vi "MainColorNoise.vi"() -> ()   [LabVIEW 2015]
panel:
  in  "Tab Control 2":T1(tab)
  in  "channel 2":cluster{"output":bool}
  in  "channel 1":T2={"Modulation Waveform (1: Sine)"=200, "modulation"=FALSE, "output"=FALSE, "Peak Deviation (90)"=90.0, "Modulation Frequency (10000)"=10000.0} {"Modulation Waveform (1: Sine)" items=["Sine"=1, "Square"=2, "Triangle"=3, "Ramp Up"=4, "Ramp Down"=5, "Noise"=100, "Arbitrary User1"=200, "Arbitrary User2"=201, "Arbitrary User3"=202, "Arbitrary User4"=203, "Edit Memory"=204]}
  in  "outpout mode":i32(ring) items=["Standard Waveform", "Arbitrary Waveform"]
  in  "configuration main":bool
  in  "amplitude (1)":dbl=0.2
  in  "dc offset (0.00)":dbl
  in  "frequency (1000000)":dbl=80000000.0
  in  "start phase (0.00)":dbl
  in  "amplitude (1) 2":dbl=0.2 caption="amplitude (1)"
  in  "dc offset (0.00) 2":dbl caption="dc offset (0.00)"
  in  "frequency (1000000) 2":dbl=80000000.0 caption="frequency (1000000)"
  in  "start phase (0.00) 2":dbl caption="start phase (0.00)"
  in  "force trigger":bool
  in  "trigger":bool
  in  "trigger source (1: External)":i32(ring)=1 items=["External"=1, "Internal"=3]
  in  "Trigger Slope (1: Positive)":i32(ring)=1 caption="external trigger Slope" items=["Positive"=1, "Negative"=2]
  in  "Output Mode (1: Trigger)":i32(ring)=1 caption="Output Mode" items=["Trigger"=1, "Sync"=2]
  in  "trigger rate (1000.0)":dbl=1000.0 caption="internal trigger rate"
  in  "trigger source (1: External) 2":i32(ring)=1 caption="trigger source (1: External)" items=["External"=1, "Internal"=3]
  in  "Burst Mode (1: Triggered)":i32(ring)=1 items=["Triggered"=1, "Gated"=2]
  in  "loading on slot 2":bool
  in  "slot (0: Slot 1) 2":i32(ring) caption="USER (0: Slot 1)" items=["Slot 1", "Slot 2", "Slot 3", "Slot 4"]
  out "waveform selected":dbl[](graph)
  in  "burst waveform":bool
  out "rep frequency":dbl
  in  "Channel Name (\"1\")":string="1"
  in  "gain (0.5) 2":dbl=0.5 caption="gain"
  out "Noise density":dbl[](graph)
  in  "slot (0: Slot 1)":i32(ring) caption="USER (0: Slot 1)" items=["Slot 1", "Slot 2", "Slot 3", "Slot 4"]
  in  "gain (0.5)":dbl=0.5
  in  "offset (0.00)":dbl
  in  "loading on channel 1":bool
  in  "Waveform Size (1000)":i32=1000
  in  "waveform generation":bool
  out "1/x":dbl
  out "min waveform size":i32
  out "max waveform size":i32
  out "waveform quantum":i32
  out "max number of waveforms":i32
  out "transfer error":errorcluster caption="error out" {"code" format="%.0x"}
  in  "resource name":refnum<k15>
  in  "Stop Button":bool
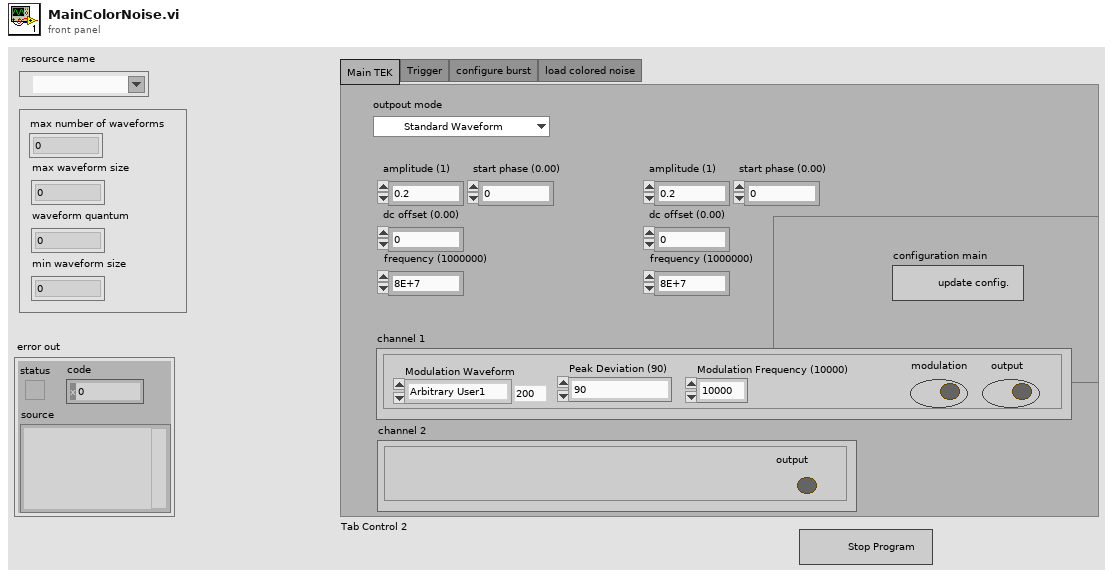
[diagram p1: front panel]
types:
  T1 = enum32{"Main TEK", "Trigger", "configure burst", "load colored noise"}
  T2 = cluster{"Modulation Waveform (1: Sine)":i32, "modulation":bool, "output":bool, "Peak Deviation (90)":dbl, "Modulation Frequency (10000)":dbl}
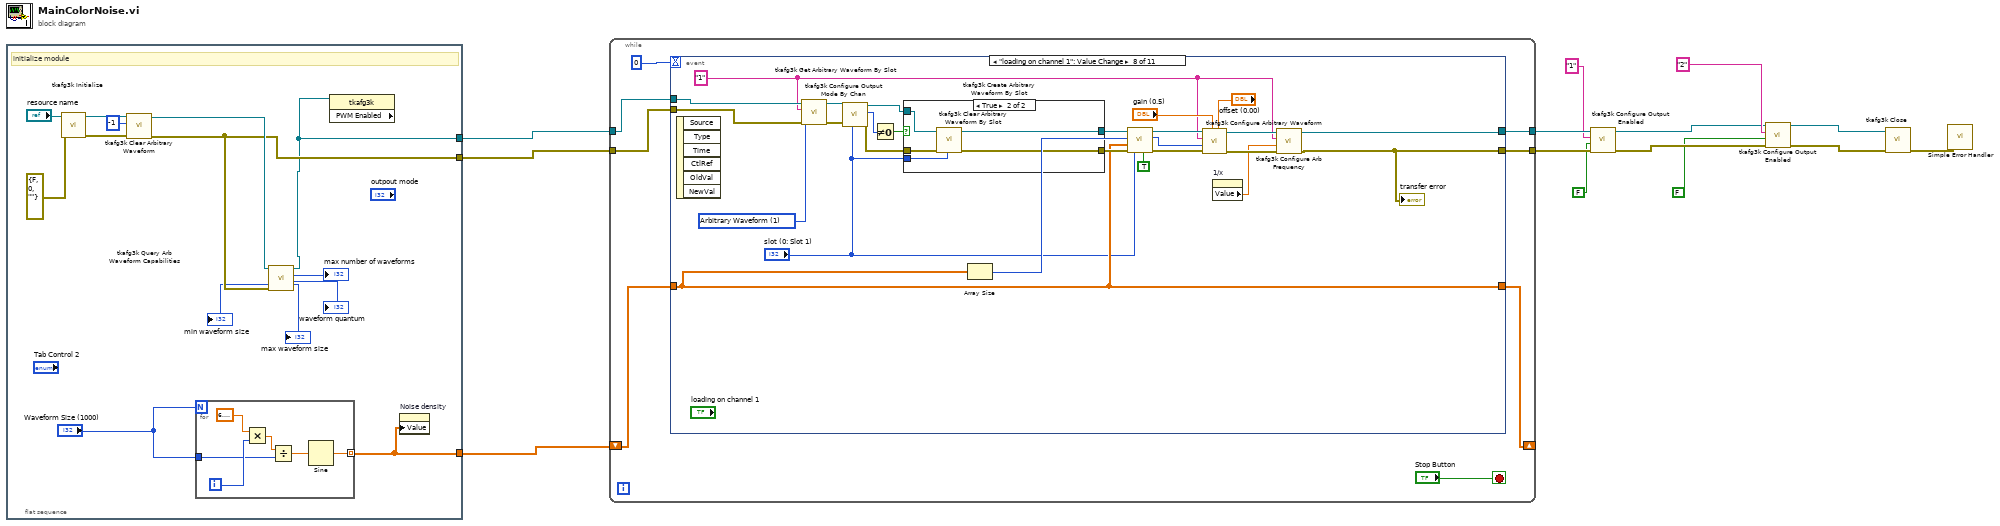
[diagram p0: block diagram]
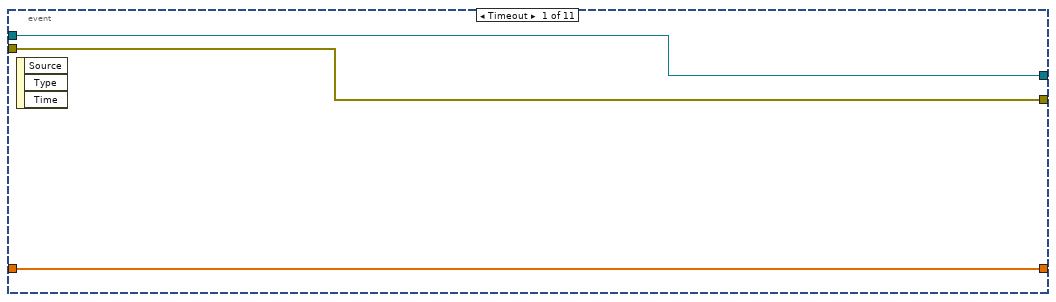
[diagram p2: hidden frame]
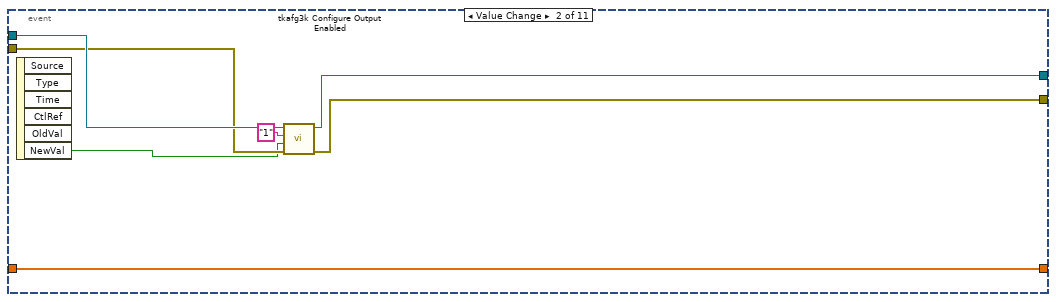
[diagram p3: hidden frame]
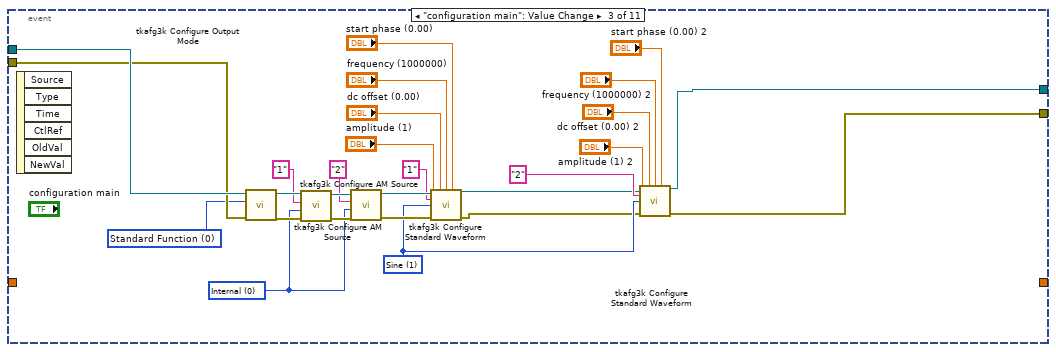
[diagram p4: hidden frame]
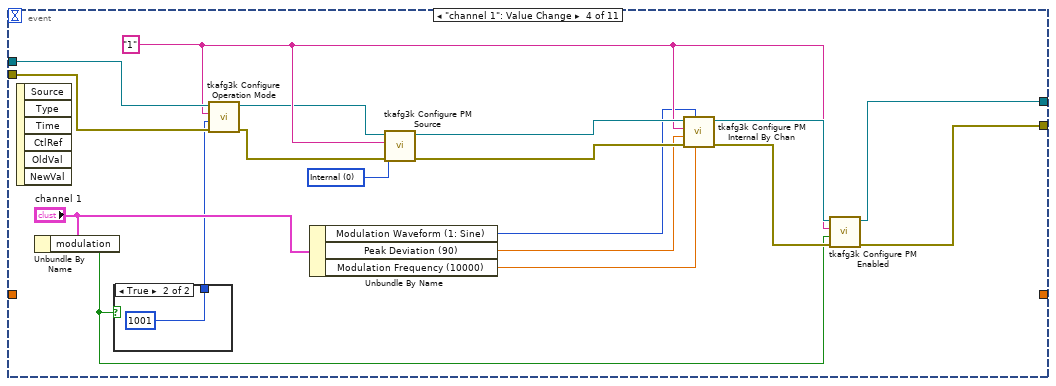
[diagram p5: hidden frame]
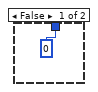
[diagram p6: hidden frame]
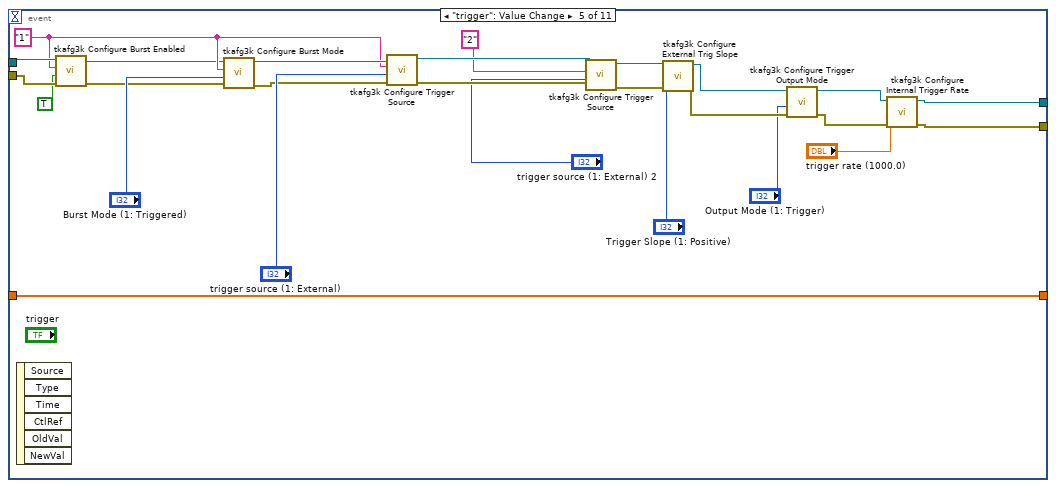
[diagram p7: hidden frame]
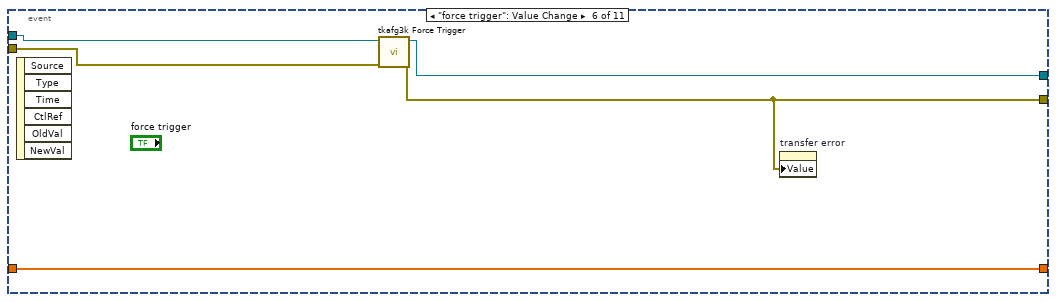
[diagram p8: hidden frame]
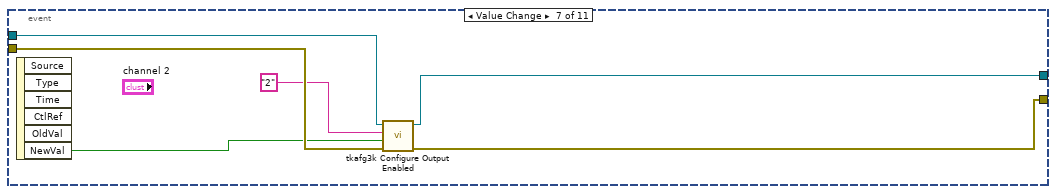
[diagram p9: hidden frame]
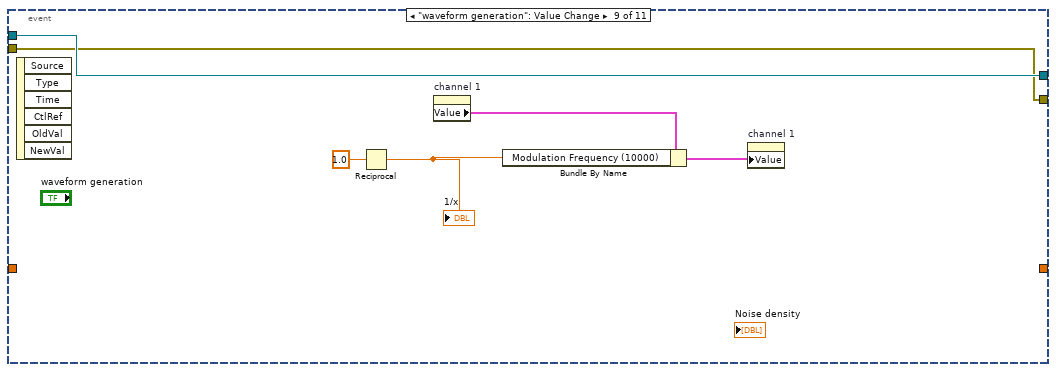
[diagram p11: hidden frame]
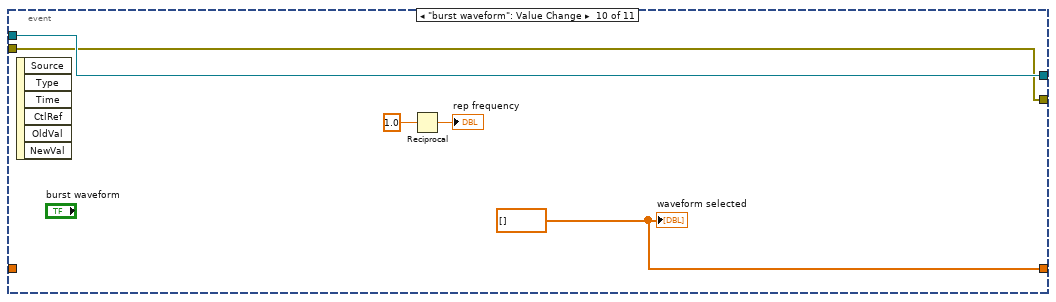
[diagram p12: hidden frame]
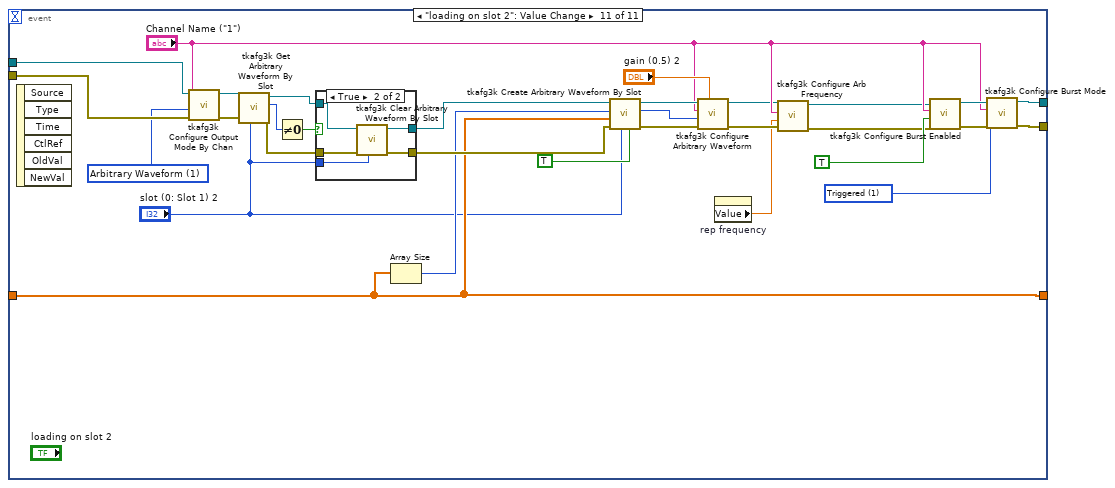
[diagram p13: hidden frame]
diagram:
  n1 = flat-sequence {
    tunnel: [w14] -> w10
    tunnel: [w22] -> w9
    tunnel: [w15] -> w5
    frame #0 {
      # "initialize module"
      n2 = call <instrlib>:"tkafg3k Initialize.vi"("error in (no error)"=errorcluster {"status"=FALSE, "code"=0, "source"=""}, "resource name"="resource name") -> ("error out"=w24:errorcluster, "instrument handle out"=w26:refnum<k15>)  [unwired: 8 in]
      n3 = call <instrlib>:"tkafg3k Clear Arbitrary Waveform.vi"("error in (no error)"=w24, "waveform handle"=-1, "instrument handle"=w26) -> ("error out"=w22:errorcluster, "instrument handle out"=w23:refnum<k15>)  [unwired: 7 in]
      n4 = for {
        N: "Waveform Size (1000)" -> [_]
        tunnel: "Waveform Size (1000)" -> [w29]
        tunnel: [w28] -> w15 mode=indexing
        i -> [w30]
        n5 = Multiply(x=6.283185307179586, y=w30) -> (x*y=w31:dbl)
        n6 = Divide(x=w31, y=w29) -> (x/y=w32:dbl)
        n7 = Sine(x=w32) -> (sin(x)=w28:dbl)
      }
      n8 = call <instrlib>:"tkafg3k Query Arb Waveform Capabilities.vi"("error in (no error)"=w22, "instrument handle"=w23) -> ("waveform quantum"=→"waveform quantum":i32, "max number of waveforms"=→"max number of waveforms":i32, "instrument handle out"=w14:refnum<k15>, "max waveform size"=→"max waveform size":i32, "min waveform size"=→"min waveform size":i32)  [unwired: 4 in, 1 out]
      n9 = property class="tkafg3k" props=["PWM Enabled"](reference=w14) -> ()  [unwired: 1 in, 3 out]
      n10 = property on="Noise density" class="WFGraph (strict)"("Value"=w15) -> ()  [unwired: 2 in, 2 out]
    }
  }
  n11 = while {
    tunnel: w10 -> [w40]
    tunnel: [w39] -> w4
    tunnel: w9 -> [w37]
    tunnel: [w36] -> w8
    shift-right: [w34] -> _
    shift-left: w5 -> [w35]
    stop <- "Stop Button" stop-if-true
    n12 = event shown="[7] \"loading on channel 1\": Value Change" {
      selector: _ -> [_ _ _ _ _ _ _ _ _ _ _]
      dyn-events: _ -> [_ _ _ _ _ _ _ _ _ _ _]
      timeout: 0 -> [_ _ _ _ _ _ _ _ _ _ _]
      tunnel: w40 -> [w43 w51 w78 w96 w104 w129 w135 w154 w174 w179 w204]
      tunnel: [w43 w50 w52 w86 w109 w127 w133 w139 w174 w179 w188] -> w39
      tunnel: w37 -> [w44 w48 w77 w95 w103 w128 w134 w153 w173 w178 w203]
      tunnel: [w44 w47 w53 w85 w108 w125 w132 w140 w173 w178 w189] -> w36
      tunnel: w35 -> [w42 w46 _ _ w124 w126 _ w149 _ _ w198]
      tunnel: [w42 w46 _ _ w124 w126 _ w149 _ w176 w198] -> w34
      event Timeout {
        n13 = event-data() -> ()  [unwired: 1 in, 3 out]
      }
      event "channel 1.output": Value Change {
        n14 = event-data() -> ("NewVal"=w45:bool)  [unwired: 1 in, 5 out]
        n15 = call <instrlib>:"tkafg3k Configure Output Enabled.vi"("error in (no error)"=w48, "channel enabled (True)"=w45, "channel name (\"1\")"="1" ("channel name (\"1\")"), "instrument handle"=w51) -> ("error out"=w47:errorcluster, "instrument handle out"=w50:refnum<k15>)  [unwired: 6 in]
      }
      event "configuration main": Value Change {
        w60 = 1 items=["Sine"=1, "Square"=2, "Pulse"=1002, "Ramp"=1001, "Noise"=1003, "DC"=6, "Sin(x)/x"=1004, "Gaussian"=1005, "Lorentz"=1006, "Exponential Rise"=1007, "Exponential Decay"=1008, "Haversine"=1009] ("waveform (1: Sine)")
        w69 = 0 items=["Internal", "External"] ("source (0: Internal)")
        w76 = 0 items=["Standard Function", "Arbitrary Waveform"] ("output mode (0: Standard Function)")
        n16 = event-data() -> ()  [unwired: 1 in, 6 out]
        n17 = call <instrlib>:"tkafg3k Configure Output Mode.vi"("error in (no error)"=w77, "output mode (0: Standard Function)"=w76, "instrument handle"=w78) -> ("error out"=w74:errorcluster, "instrument handle out"=w75:refnum<k15>)  [unwired: 7 in]
        n18 = call <instrlib>:"tkafg3k Configure AM Source.vi"("error in (no error)"=w74, "source (0: Internal)"=w69, "channel name (\"1\")"="1" ("channel name (\"1\")"), "instrument handle"=w75) -> ("error out"=w73:errorcluster, "instrument handle out"=w72:refnum<k15>)  [unwired: 6 in]
        n19 = call <instrlib>:"tkafg3k Configure AM Source.vi"("error in (no error)"=w73, "source (0: Internal)"=w69, "channel name (\"1\")"="2" ("channel name (\"1\")"), "instrument handle"=w72) -> ("error out"=w66:errorcluster, "instrument handle out"=w68:refnum<k15>)  [unwired: 6 in]
        n20 = call <instrlib>:"tkafg3k Configure Standard Waveform.vi"("instrument handle"=w68, "dc offset (0.00)"="dc offset (0.00)", "frequency (1000000)"="frequency (1000000)", "start phase (0.00)"="start phase (0.00)", "channel name (\"1\")"="1" ("channel name (\"1\")"), "waveform (1: Sine)"=w60, "amplitude (1)"="amplitude (1)", "error in (no error)"=w66) -> ("instrument handle out"=w58:refnum<k15>, "error out"=w59:errorcluster)  [unwired: 6 in]
        n21 = call <instrlib>:"tkafg3k Configure Standard Waveform.vi"("instrument handle"=w58, "dc offset (0.00)"="dc offset (0.00) 2", "frequency (1000000)"="frequency (1000000) 2", "start phase (0.00)"="start phase (0.00) 2", "channel name (\"1\")"="2" ("channel name (\"1\")"), "waveform (1: Sine)"=w60, "amplitude (1)"="amplitude (1) 2", "error in (no error)"=w59) -> ("instrument handle out"=w52:refnum<k15>, "error out"=w53:errorcluster)  [unwired: 6 in]
      }
      event "channel 1": Value Change {
        w94 = 0 items=["Internal", "External"] ("Source (0: Internal)")
        w88 = "1" ("channel name (\"1\")")
        n22 = event-data() -> ()  [unwired: 1 in, 6 out]
        n23 = Unbundle By Name("channel 1") -> ("modulation"=w79:bool)
        n24 = case shown="True" w79 {
          tunnel: [0 ("operation mode channel 3") 1001 ("operation mode channel 3")] -> w80
          frame False {
          }
          frame True {
          }
        }
        n25 = call <instrlib>:"tkafg3k Configure Operation Mode.vi"("error in (no error)"=w95, "operation mode (0: Continuous)"=w80, "channel name (\"1\")"=w88, "instrument handle"=w96) -> ("error out"=w93:errorcluster, "instrument handle out"=w87:refnum<k15>)  [unwired: 6 in]
        n26 = Unbundle By Name("channel 1") -> ("Modulation Waveform (1: Sine)"=w84:i32, "Peak Deviation (90)"=w82:dbl, "Modulation Frequency (10000)"=w81:dbl)
        n27 = call <instrlib>:"tkafg3k Configure PM Source.vi"("error in (no error)"=w93, "Source (0: Internal)"=w94, "Channel Name (\"1\")"=w88, "instrument handle"=w87) -> ("error out"=w91:errorcluster, "instrument handle out"=w92:refnum<k15>)  [unwired: 6 in]
        n28 = call <instrlib>:"tkafg3k Configure PM Internal By Chan.vi"("Modulation Frequency (10000)"=w81, "Modulation Waveform (1: Sine)"=w84, "error in (no error)"=w91, "Peak Deviation (90)"=w82, "Channel Name (\"1\")"=w88, "instrument handle"=w92) -> ("error out"=w89:errorcluster, "instrument handle out"=w90:refnum<k15>)  [unwired: 4 in]
        n29 = call <instrlib>:"tkafg3k Configure PM Enabled.vi"("error in (no error)"=w89, "Enabled (True)"=w79, "Channel Name (\"1\")"=w88, "instrument handle"=w90) -> ("error out"=w85:errorcluster, "instrument handle out"=w86:refnum<k15>)  [unwired: 6 in]
      }
      event "trigger": Value Change {
        w102 = "1" ("channel name (\"1\")")
        n30 = event-data() -> ()  [unwired: 1 in, 6 out]
        n31 = call <instrlib>:"tkafg3k Configure Burst Enabled.vi"("error in (no error)"=w103, "Burst Enabled (True)"=TRUE, "Channel Name (\"1\")"=w102, "instrument handle"=w104) -> ("error out"=w99:errorcluster, "instrument handle out"=w100:refnum<k15>)  [unwired: 6 in]
        n32 = call <instrlib>:"tkafg3k Configure Burst Mode.vi"("error in (no error)"=w99, "Burst Mode (1: Triggered)"="Burst Mode (1: Triggered)", "Channel Name (\"1\")"=w102, "instrument handle"=w100) -> ("error out"=w107:errorcluster, "instrument handle out"=w106:refnum<k15>)  [unwired: 6 in]
        n33 = call <instrlib>:"tkafg3k Configure Trigger Source.vi"("error in (no error)"=w107, "trigger source (1: External)"="trigger source (1: External)", "channel name (\"1\")"=w102, "instrument handle"=w106) -> ("error out"=w120:errorcluster, "instrument handle out"=w122:refnum<k15>)  [unwired: 6 in]
        n34 = call <instrlib>:"tkafg3k Configure Trigger Source.vi"("error in (no error)"=w120, "trigger source (1: External)"="trigger source (1: External) 2", "channel name (\"1\")"="2" ("channel name (\"1\")"), "instrument handle"=w122) -> ("error out"=w117:errorcluster, "instrument handle out"=w118:refnum<k15>)  [unwired: 6 in]
        n35 = call <instrlib>:"tkafg3k Configure External Trig Slope.vi"("error in (no error)"=w117, "Trigger Slope (1: Positive)"="Trigger Slope (1: Positive)", "instrument handle"=w118) -> ("error out"=w114:errorcluster, "instrument handle out"=w115:refnum<k15>)  [unwired: 7 in]
        n36 = call <instrlib>:"tkafg3k Configure Trigger Output Mode.vi"("error in (no error)"=w114, "Output Mode (1: Trigger)"="Output Mode (1: Trigger)", "instrument handle"=w115) -> ("error out"=w111:errorcluster, "instrument handle out"=w112:refnum<k15>)  [unwired: 7 in]
        n37 = call <instrlib>:"tkafg3k Configure Internal Trigger Rate.vi"("error in (no error)"=w111, "trigger rate (1000.0)"="trigger rate (1000.0)", "instrument handle"=w112) -> ("error out"=w108:errorcluster, "instrument handle out"=w109:refnum<k15>)  [unwired: 7 in]
      }
      event "force trigger": Value Change {
        n38 = event-data() -> ()  [unwired: 1 in, 6 out]
        n39 = call <instrlib>:"tkafg3k Force Trigger.vi"("error in (no error)"=w128, "instrument handle"=w129) -> ("error out"=w125:errorcluster, "instrument handle out"=w127:refnum<k15>)  [unwired: 8 in]
        n40 = property on="transfer error" class="Clust (strict)"("Value"=w125) -> ()  [unwired: 2 in, 2 out]
      }
      event "channel 2.output": Value Change {
        n41 = event-data() -> ("NewVal"=w130:bool)  [unwired: 1 in, 5 out]
        n42 = call <instrlib>:"tkafg3k Configure Output Enabled.vi"("error in (no error)"=w134, "channel enabled (True)"=w130, "channel name (\"1\")"="2" ("channel name (\"1\")"), "instrument handle"=w135) -> ("error out"=w132:errorcluster, "instrument handle out"=w133:refnum<k15>)  [unwired: 6 in]
      }
      event "loading on channel 1": Value Change {
        w161 = 1 items=["Standard Function", "Arbitrary Waveform"] ("Output Mode (0: Standard Function)")
        w137 = "1" ("Channel Name (\"1\")")
        n43 = event-data() -> ()  [unwired: 1 in, 6 out]
        n44 = call <instrlib>:"tkafg3k Configure Output Mode By Chan.vi"("error in (no error)"=w153, "Output Mode (0: Standard Function)"=w161, "Channel Name (\"1\")"=w137, "instrument handle"=w154) -> ("error out"=w159:errorcluster, "instrument handle out"=w160:refnum<k15>)  [unwired: 6 in]
        n45 = call <instrlib>:"tkafg3k Get Arbitrary Waveform By Slot.vi"("slot (0: Slot 1)"="slot (0: Slot 1)", "error in (no error)"=w159, "instrument handle"=w160) -> ("error out"=w158:errorcluster, "waveform handle"=w155:i32, "instrument handle out"=w157:refnum<k15>)  [unwired: 6 in]
        n46 = Not Equal To 0?(x=w155) -> (x != 0?=w156:bool)
        n47 = case shown="True" w156 {
          tunnel: w157 -> [w163 w168]
          tunnel: w158 -> [w162 w167]
          tunnel: [w163 w166] -> w152
          tunnel: [w162 w165] -> w151
          tunnel: "slot (0: Slot 1)" -> [_ w164]
          frame False {
          }
          frame True {
            n48 = call <instrlib>:"tkafg3k Clear Arbitrary Waveform By Slot.vi"("slot (0: Slot 1)"=w164, "error in (no error)"=w167, "instrument handle"=w168) -> ("error out"=w165:errorcluster, "instrument handle out"=w166:refnum<k15>)  [unwired: 7 in]
          }
        }
        n49 = Array Size(array=w149) -> (size(s)=w150:i32)
        n50 = call <instrlib>:"tkafg3k Create Arbitrary Waveform By Slot.vi"("overwrite (False)"=TRUE, "slot (0: Slot 1)"="slot (0: Slot 1)", "error in (no error)"=w151, "waveform data array"=w149, "waveform size (1000)"=w150, "instrument handle"=w152) -> ("error out"=w145:errorcluster, "waveform handle"=w146:i32, "instrument handle out"=w147:refnum<k15>)  [unwired: 3 in]
        n51 = call <instrlib>:"tkafg3k Configure Arbitrary Waveform.vi"("offset (0.00)"="offset (0.00)", "gain (0.5)"="gain (0.5)", "error in (no error)"=w145, "waveform handle"=w146, "channel name (\"1\")"=w137, "instrument handle"=w147) -> ("error out"=w141:errorcluster, "instrument handle out"=w138:refnum<k15>)  [unwired: 4 in]
        n52 = property on="1/x" class="DigNum (strict)"() -> ("Value"=w136:dbl)  [unwired: 2 in, 2 out]
        n53 = call <instrlib>:"tkafg3k Configure Arb Frequency.vi"("error in (no error)"=w141, "frequency (1000000)"=w136, "channel name (\"1\")"=w137, "instrument handle"=w138) -> ("error out"=w140:errorcluster, "instrument handle out"=w139:refnum<k15>)  [unwired: 6 in]
        "transfer error" <- w140
      }
      event "waveform generation": Value Change {
        n54 = event-data() -> ()  [unwired: 1 in, 6 out]
        n55 = Reciprocal(x=1.0) -> (1/x=w171:dbl)
        "1/x" <- w171
        n56 = property on="channel 1" class="Clust (strict)"() -> ("Value"=w172:T2)  [unwired: 2 in, 2 out]
        n57 = Bundle By Name(cluster=w172, "Modulation Frequency (10000)"=w171) -> (w170:T2)
        n58 = property on="channel 1" class="Clust (strict)"("Value"=w170) -> ()  [unwired: 2 in, 2 out]
      }
      event "burst waveform": Value Change {
        w176 = dbl[] [] ("waveform selected")
        n59 = event-data() -> ()  [unwired: 1 in, 6 out]
        n60 = Reciprocal(x=1.0) -> (1/x=→"rep frequency":dbl)
        "waveform selected" <- w176
      }
      event "loading on slot 2": Value Change {
        w187 = 1 items=["Triggered"=1, "Gated"=2] ("Burst Mode (1: Triggered)")
        w202 = 1 items=["Standard Function", "Arbitrary Waveform"] ("Output Mode (0: Standard Function)")
        n61 = event-data() -> ()  [unwired: 1 in, 6 out]
        n62 = call <instrlib>:"tkafg3k Configure Output Mode By Chan.vi"("error in (no error)"=w203, "Output Mode (0: Standard Function)"=w202, "Channel Name (\"1\")"="Channel Name (\"1\")", "instrument handle"=w204) -> ("error out"=w206:errorcluster, "instrument handle out"=w205:refnum<k15>)  [unwired: 6 in]
        n63 = call <instrlib>:"tkafg3k Get Arbitrary Waveform By Slot.vi"("slot (0: Slot 1)"="slot (0: Slot 1) 2", "error in (no error)"=w206, "instrument handle"=w205) -> ("error out"=w207:errorcluster, "waveform handle"=w210:i32, "instrument handle out"=w208:refnum<k15>)  [unwired: 6 in]
        n64 = Not Equal To 0?(x=w210) -> (x != 0?=w209:bool)
        n65 = case shown="True" w209 {
          tunnel: w208 -> [w212 w217]
          tunnel: w207 -> [w211 w216]
          tunnel: [w212 w215] -> w201
          tunnel: [w211 w214] -> w200
          tunnel: "slot (0: Slot 1) 2" -> [_ w213]
          frame False {
          }
          frame True {
            n66 = call <instrlib>:"tkafg3k Clear Arbitrary Waveform By Slot.vi"("slot (0: Slot 1)"=w213, "error in (no error)"=w216, "instrument handle"=w217) -> ("error out"=w214:errorcluster, "instrument handle out"=w215:refnum<k15>)  [unwired: 7 in]
          }
        }
        n67 = Array Size(array=w198) -> (size(s)=w199:i32)
        n68 = call <instrlib>:"tkafg3k Create Arbitrary Waveform By Slot.vi"("overwrite (False)"=TRUE, "slot (0: Slot 1)"="slot (0: Slot 1) 2", "error in (no error)"=w200, "waveform data array"=w198, "waveform size (1000)"=w199, "instrument handle"=w201) -> ("error out"=w195:errorcluster, "waveform handle"=w196:i32, "instrument handle out"=w197:refnum<k15>)  [unwired: 3 in]
        n69 = call <instrlib>:"tkafg3k Configure Arbitrary Waveform.vi"("gain (0.5)"="gain (0.5) 2", "error in (no error)"=w195, "waveform handle"=w196, "channel name (\"1\")"="Channel Name (\"1\")", "instrument handle"=w197) -> ("error out"=w185:errorcluster, "instrument handle out"=w182:refnum<k15>)  [unwired: 5 in]
        n70 = property on="rep frequency" class="DigNum (strict)"() -> ("Value"=w180:dbl)  [unwired: 2 in, 2 out]
        n71 = call <instrlib>:"tkafg3k Configure Arb Frequency.vi"("error in (no error)"=w185, "frequency (1000000)"=w180, "channel name (\"1\")"="Channel Name (\"1\")", "instrument handle"=w182) -> ("error out"=w184:errorcluster, "instrument handle out"=w181:refnum<k15>)  [unwired: 6 in]
        n72 = call <instrlib>:"tkafg3k Configure Burst Enabled.vi"("error in (no error)"=w184, "Burst Enabled (True)"=TRUE, "Channel Name (\"1\")"="Channel Name (\"1\")", "instrument handle"=w181) -> ("error out"=w191:errorcluster, "instrument handle out"=w190:refnum<k15>)  [unwired: 6 in]
        n73 = call <instrlib>:"tkafg3k Configure Burst Mode.vi"("error in (no error)"=w191, "Burst Mode (1: Triggered)"=w187, "Channel Name (\"1\")"="Channel Name (\"1\")", "instrument handle"=w190) -> ("error out"=w189:errorcluster, "instrument handle out"=w188:refnum<k15>)  [unwired: 6 in]
      }
    }
  }
  n74 = call <instrlib>:"tkafg3k Configure Output Enabled.vi"("channel enabled (True)"=FALSE, "channel name (\"1\")"="1" ("channel name (\"1\")"), "instrument handle"=w4) -> ("instrument handle out"=w3:refnum<k15>)  [unwired: 7 in, 1 out]
  n75 = call <instrlib>:"tkafg3k Configure Output Enabled.vi"("error in (no error)"=w8, "channel enabled (True)"=FALSE, "channel name (\"1\")"="2" ("channel name (\"1\")"), "instrument handle"=w3) -> ("error out"=w13:errorcluster, "instrument handle out"=w12:refnum<k15>)  [unwired: 6 in]
  n76 = call <instrlib>:"tkafg3k Close.vi"("error in (no error)"=w13, "instrument handle"=w12) -> ("error out"=w11:errorcluster)  [unwired: 9 in]
  n77 = call <vilib>:"Simple Error Handler.vi"("error in (no error)"=w11) -> ()  [unwired: 1 in, 8 out]
